vi "Init Hardware.vi"(8 "error in (no error)":errorcluster, 11 "Tektronix Driver in":refnum<class "Tektronix 7000 Driver.lvclass">) -> (0 "error out":errorcluster, 3 "Tektronix Driver out":refnum<class "Tektronix 7000 Driver.lvclass">)   [LabVIEW 2020, in "Tektronix 7000 Driver.lvclass"]
uses:
  Tektronix 7000 Driver.lvclass
  C:/GitHub/NHMFL_Core/Libraries/Instruments/Tektronix/Tektronix Driver/Tektronix Driver.lvclass
  <instrlib>/Tektronix 7000 Series/Tektronix 7000 Series.lvlib
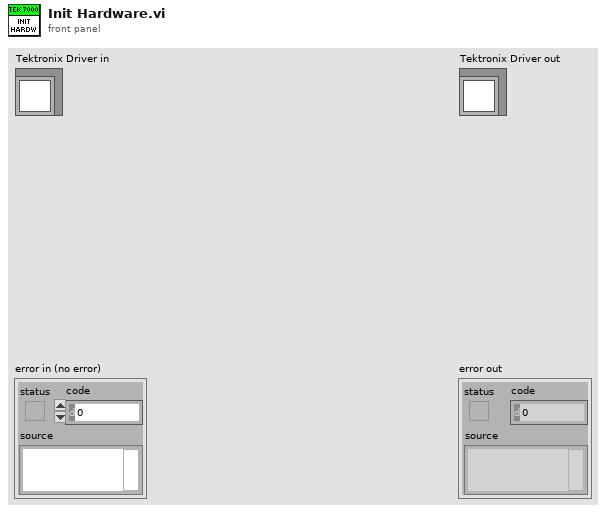
[diagram p1: front panel]
types:
  T1 = typedef "Tektronix Configuration.ctl" = cluster{"Channel":i32, "Number of averages":i32, "Input impedace":enum16{"1 M Ohm", "50 Ohm"}, "Vertical coupling":enum16{"AC", "DC", "Ground"}}
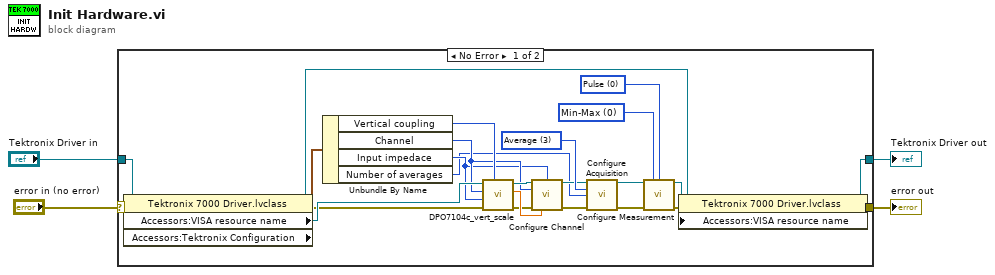
[diagram p0: block diagram]
diagram:
  n1 = case shown="No Error" "error in (no error)" {
    selector: "error in (no error)" -> [w28 w30]
    tunnel: [w8 w30] -> w3
    tunnel: [w6 w29] -> w1
    tunnel: "Tektronix Driver in" -> [w27 w29]
    frame No Error {
      w10 = u16 0 items=["Min-Max", "Histogram", "Histogram Mean"] ("Ref Level Calculate Method (1:Histogram)")
      w11 = u16 0 items=["Pulse", "Eye"] ("Signal Type (0:Pulse)")
      w16 = u16 3 items=["Sample", "Peak Detect", "Hi Res", "Average", "Envelope", "WfmDB"] ("Acquisition Type (0:Sample)")
      n2 = property class="Tektronix 7000 Driver.lvclass"(reference=w27, error in=w28) -> (reference out=w7:refnum<class "Tektronix 7000 Driver.lvclass">, error out=w24:errorcluster, "Accessors:VISA resource name"=w26:refnum<visa-resource-name>, "Accessors:Tektronix Configuration"=w25:T1)
      n3 = Unbundle By Name(w25) -> ("Vertical coupling"=w23:enum16{"AC", "DC", "Ground"}, "Channel"=w19:i32, "Input impedace"=w18:enum16{"1 M Ohm", "50 Ohm"}, "Number of averages"=w14:i32)
      n4 = call "DPO7104c_vert_scale.vi"("Vertical Coupling (1: DC)"=w23, "error in (no error)"=w24, "Input Impedance (0: 1M ohm)"=w18, "Channel (0: Channel 1)"=w19, "VISA resource name"=w26) -> ("error out"=w21:errorcluster, "vertical range"=w22:dbl, "VISA resource name out"=w20:refnum<visa-resource-name>)  [unwired: 4 in]
      n5 = call <instrlib>:"Configure Channel.vi"("VISA resource name"=w20, "Input Impedance (0: 1M ohm)"=w18, "Channel (0: Channel 1)"=w19, "error in (no error)"=w21, "Vertical Range (10.0 V)"=w22) -> ("VISA resource name out"=w15:refnum<visa-resource-name>, "error out"=w17:errorcluster)  [unwired: 9 in]
      n6 = call <instrlib>:"Configure Acquisition.vi"("VISA resource name"=w15, "Acquisition Type (0:Sample)"=w16, "Average Waveforms (10)"=w14, "error in (no error)"=w17) -> ("VISA resource name out"=w12:refnum<visa-resource-name>, "error out"=w13:errorcluster)  [unwired: 10 in]
      n7 = call <instrlib>:"Configure Measurement.vi"("VISA resource name"=w12, "Ref Level Calculate Method (1:Histogram)"=w10, "Signal Type (0:Pulse)"=w11, "error in (no error)"=w13) -> ("VISA resource name out"=w5:refnum<visa-resource-name>, "error out"=w9:errorcluster)  [unwired: 10 in]
      n8 = property class="Tektronix 7000 Driver.lvclass"(reference=w7, error in=w9, "Accessors:VISA resource name"=w5) -> (reference out=w6:refnum<class "Tektronix 7000 Driver.lvclass">, error out=w8:errorcluster)
    }
    frame Error {
    }
  }
  "error out" <- w3
  "Tektronix Driver out" <- w1
